vi "Get_radio_info.vi"(6 "VISA resource name":refnum<visa-resource-name>="COM5", 8 "error in (no error)":errorcluster, 9 "RadioType":T2) -> (0 "error out":errorcluster, 2 "Software Package Lines":string, 3 "Radio info":T1, 4 "VISA resource name out":refnum<visa-resource-name>)   [LabVIEW 2024]
uses:
  MTCDT_radio_type.ctl
panel:
  out "rssi":string
  out "rsrp":string
  out "rsrq":string
  out "Response Line 5":string
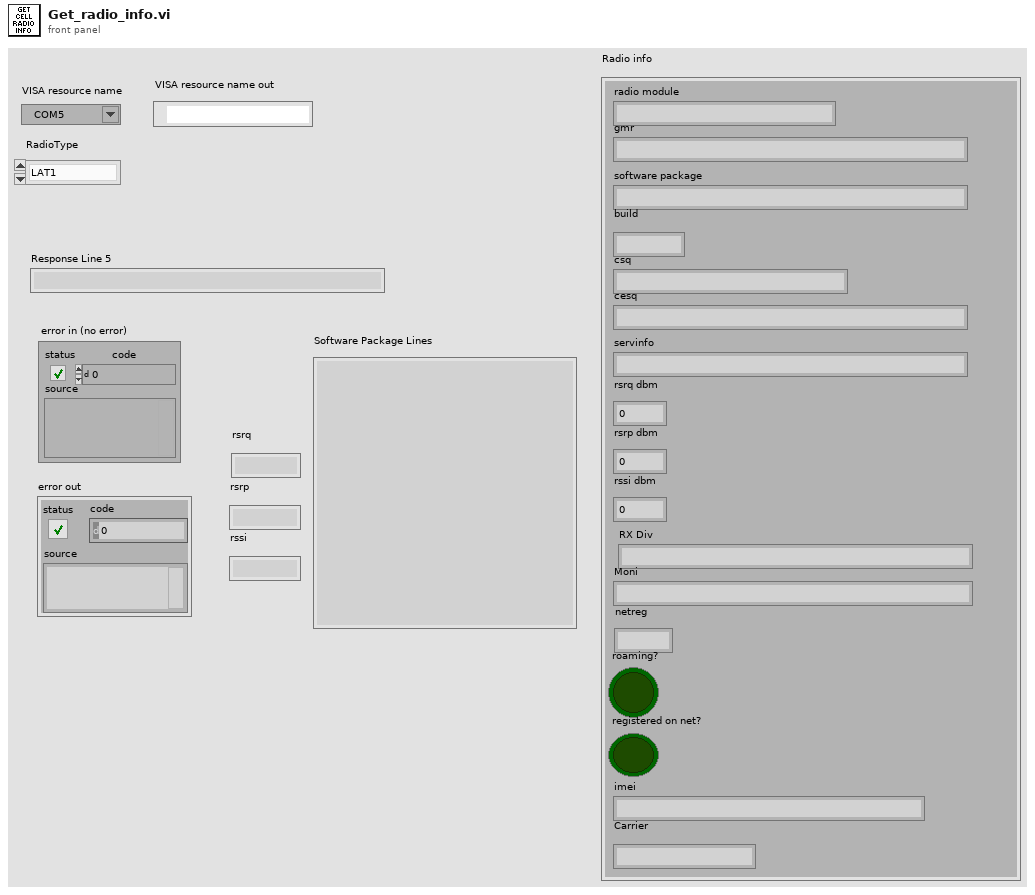
[diagram p1: front panel]
types:
  T1 = cluster{"radio module":string, "gmr":string, "software package":string, "csq":string, "cesq":string, "servinfo":string, "rsrq dbm":dbl, "rsrp dbm":dbl, "rssi dbm":dbl, "build":string, "RX Div":string, "Moni":string, "netreg":string, "roaming?":bool, "registered on net?":bool, "imei":string, "Carrier":string}
  T2 = typedef "MTCDT_radio_type.ctl" = enum16{"LAT1", "H5", "LAT3", "LEU1", "L4E1", "L4N1", "LVW2", "LSB3", "LDC3", "LAP3", "L4G1", "L6G1"}
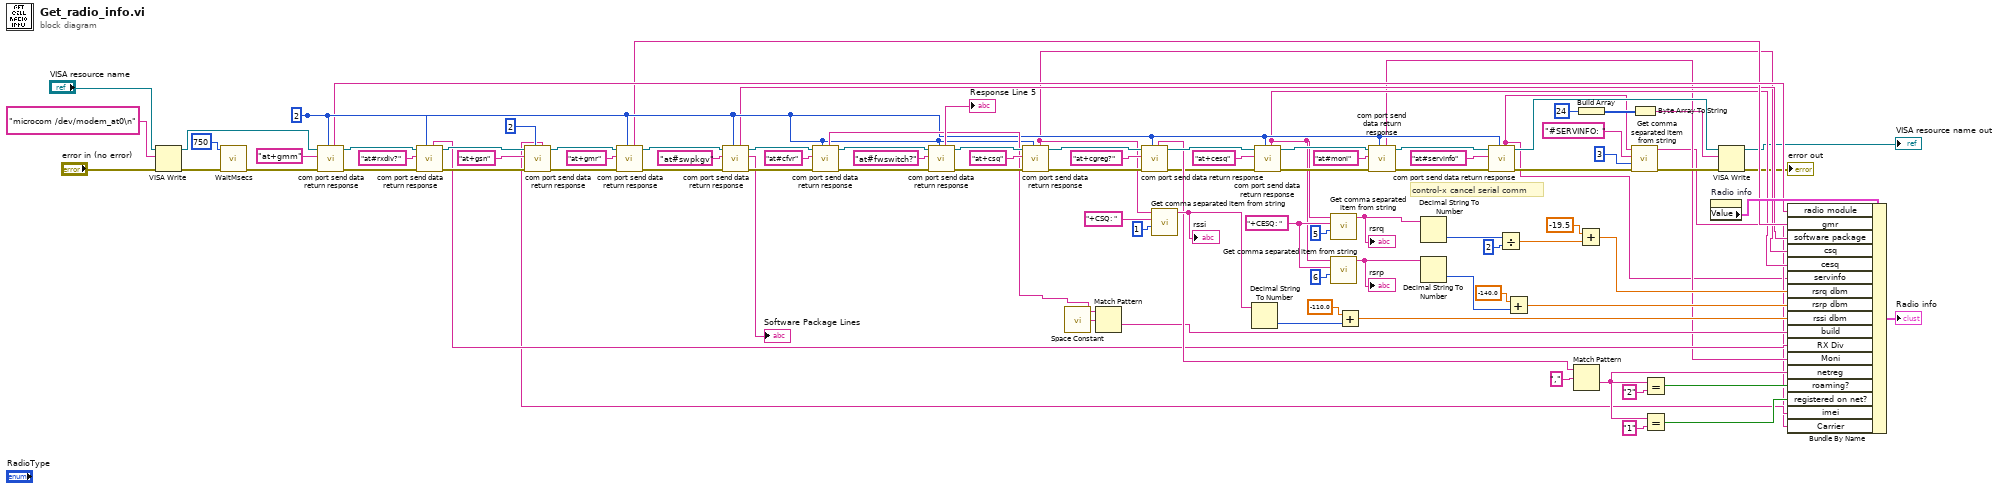
[diagram p0: block diagram]
diagram:
  w65 = "+CESQ: " ("regular expression")
  w36 = u32 2 ("Return line number")
  # "control-x cancel serial comm"
  n1 = VISA Write(VISA resource name="VISA resource name", write buffer="microcom /dev/modem_at0\n", error in (no error)="error in (no error)") -> (VISA resource name out=w70:refnum<visa-resource-name>, error out=w69:errorcluster)  [unwired: 1 out]
  n2 = call "WaitMsecs.vi"("error in (no error)"=w69, "Wait Msecs"=u32 750) -> ("error out"=w67:errorcluster)  [unwired: 9 in]
  n3 = call "com port send data return response.vi"("Return line number"=w36, "error in (no error)"=w67, "Send data"="at+gmm", "VISA resource name"=w70) -> ("error out"=w41:errorcluster, "VISA resource name out"=w44:refnum<visa-resource-name>, "Response Line"=w22:string)  [unwired: 3 in, 2 out]
  n4 = call "com port send data return response.vi"("Return line number"=w36, "error in (no error)"=w41, "Send data"="at#rxdiv?", "VISA resource name"=w44) -> ("error out"=w40:errorcluster, "VISA resource name out"=w43:refnum<visa-resource-name>, "Response Line"=w13:string)  [unwired: 3 in, 2 out]
  n5 = call "com port send data return response.vi"("Return line number"=u32 2, "error in (no error)"=w40, "Send data"="at+gsn", "VISA resource name"=w43) -> ("error out"=w49:errorcluster, "VISA resource name out"=w47:refnum<visa-resource-name>, "Response Line"=w8:string)  [unwired: 3 in, 2 out]
  n6 = call "com port send data return response.vi"("Return line number"=w36, "error in (no error)"=w49, "Send data"="at+gmr", "VISA resource name"=w47) -> ("error out"=w94:errorcluster, "VISA resource name out"=w93:refnum<visa-resource-name>, "Response Line"=w21:string)  [unwired: 3 in, 2 out]
  n7 = call "com port send data return response.vi"("Return line number"=w36, "error in (no error)"=w94, "Send data"="at#swpkgv", "VISA resource name"=w93) -> ("error out"=w91:errorcluster, "response"=→"Software Package Lines":string, "VISA resource name out"=w90:refnum<visa-resource-name>, "Response Line"=w20:string)  [unwired: 3 in, 1 out]
  n8 = call "com port send data return response.vi"("Return line number"=w36, "error in (no error)"=w91, "Send data"="at#cfvr", "VISA resource name"=w90) -> ("error out"=w88:errorcluster, "VISA resource name out"=w87:refnum<visa-resource-name>, "Response Line"=w46:string)  [unwired: 3 in, 2 out]
  n9 = call "com port send data return response.vi"("Return line number"=w36, "error in (no error)"=w88, "Send data"="at#fwswitch?", "VISA resource name"=w87) -> ("error out"=w83:errorcluster, "VISA resource name out"=w84:refnum<visa-resource-name>, "Response Line"=→"Response Line 5":string)  [unwired: 3 in, 2 out]
  n10 = call "com port send data return response.vi"("Return line number"=w36, "error in (no error)"=w83, "Send data"="at+csq", "VISA resource name"=w84) -> ("error out"=w31:errorcluster, "VISA resource name out"=w38:refnum<visa-resource-name>, "Response Line"=w19:string)  [unwired: 3 in, 2 out]
  n11 = call <vilib>:"Space Constant.vi"() -> ("String"=w45:string)
  n12 = Match Pattern(string=w46, regular expression=w45) -> (after substring=w14:string)  [unwired: 1 in, 3 out]
  n13 = call "com port send data return response.vi"("Return line number"=w36, "error in (no error)"=w31, "Send data"="at+cgreg?", "VISA resource name"=w38) -> ("error out"=w30:errorcluster, "VISA resource name out"=w37:refnum<visa-resource-name>, "Response Line"=w35:string)  [unwired: 3 in, 2 out]
  n14 = call "Get comma separated item from string.vi"("Field Num (1-n)"=u32 1, "Preamble to first item"="+CSQ: ", "String to parse with commas"=w19) -> ("Item string value"=w61:string)  [unwired: 7 in, 1 out]
  "rssi" <- w61
  n15 = Decimal String To Number(string=w61) -> (number=w59:i32)  [unwired: 2 in, 1 out]
  n16 = call "com port send data return response.vi"("Return line number"=w36, "error in (no error)"=w30, "Send data"="at+cesq", "VISA resource name"=w37) -> ("error out"=w80:errorcluster, "VISA resource name out"=w79:refnum<visa-resource-name>, "Response Line"=w18:string)  [unwired: 3 in, 2 out]
  n17 = call "Get comma separated item from string.vi"("Field Num (1-n)"=u32 5, "Preamble to first item"=w65, "String to parse with commas"=w18) -> ("Item string value"=w55:string)  [unwired: 7 in, 1 out]
  "rsrq" <- w55
  n18 = call "Get comma separated item from string.vi"("Field Num (1-n)"=u32 6, "Preamble to first item"=w65, "String to parse with commas"=w18) -> ("Item string value"=w58:string)  [unwired: 7 in, 1 out]
  "rsrp" <- w58
  n19 = Add(x=-110.0, y=w59) -> (x+y=w15:dbl)
  n20 = call "com port send data return response.vi"("Return line number"=w36, "error in (no error)"=w80, "Send data"="at#moni", "VISA resource name"=w79) -> ("error out"=w77:errorcluster, "VISA resource name out"=w76:refnum<visa-resource-name>, "Response Line"=w12:string)  [unwired: 3 in, 2 out]
  n21 = Decimal String To Number(string=w55) -> (number=w54:i32)  [unwired: 2 in, 1 out]
  n22 = Decimal String To Number(string=w58) -> (number=w56:i32)  [unwired: 2 in, 1 out]
  n23 = call "com port send data return response.vi"("Return line number"=w36, "error in (no error)"=w77, "Send data"="at#servinfo", "VISA resource name"=w76) -> ("error out"=w27:errorcluster, "VISA resource name out"=w25:refnum<visa-resource-name>, "Response Line"=w6:string)  [unwired: 3 in, 2 out]
  n24 = Divide(x=w54, y=2) -> (x/y=w51:dbl)
  n25 = Add(x=-140.0, y=w56) -> (x+y=w16:dbl)
  n26 = Match Pattern(string=w35, regular expression=",") -> (after substring=w11:string)  [unwired: 1 in, 3 out]
  n27 = Add(x=-19.5, y=w51) -> (x+y=w17:dbl)
  n28 = Build Array(u8 24 ("element")) -> (w73:u8[])
  n29 = call "Get comma separated item from string.vi"("error in (no error)"=w27, "Field Num (1-n)"=u32 3, "Preamble to first item"="#SERVINFO: " ("regular expression"), "String to parse with commas"=w6) -> ("error out"=w26:errorcluster, "Item string value"=w7:string)  [unwired: 6 in]
  n30 = Byte Array To String(unsigned byte array=w73) -> (string=w72:string)
  n31 = Equal?(x=w11, y="2") -> (x = y?=w9:bool)
  n32 = Equal?(x=w11, y="1") -> (x = y?=w10:bool)
  n33 = property on="Radio info" class="Clust (strict)"() -> ("Value"=w24:T1)  [unwired: 2 in, 2 out]
  n34 = VISA Write(VISA resource name=w25, write buffer=w72, error in (no error)=w26) -> (VISA resource name out=→"VISA resource name out":refnum<visa-resource-name>, error out=→"error out":errorcluster)  [unwired: 1 out]
  n35 = Bundle By Name(cluster=w24, "radio module"=w22, "gmr"=w21, "software package"=w20, "csq"=w19, "cesq"=w18, "servinfo"=w6, "rsrq dbm"=w17, "rsrp dbm"=w16, "rssi dbm"=w15, "build"=w14, "RX Div"=w13, "Moni"=w12, "netreg"=w11, "roaming?"=w9, "registered on net?"=w10, "imei"=w8, "Carrier"=w7) -> (→"Radio info":T1)
